vi "Set_Joint_State_Publlish_Rate.vi"(5 "node":string, 6 "error in":errorcluster, 9 "Publish Rate":u32) -> (0 "error out":errorcluster)   [LabVIEW 2013]
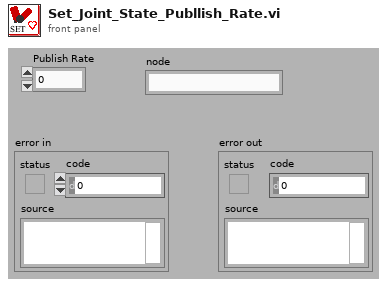
[diagram p1: front panel]
types:
  T1 = enum16{"big-endian, network order", "native, host order", "little-endian"}
  T2 = typedef "_ROSControl.ctl" = cluster{"topic port":u16, "Node":string, "topic":string, "type":string, "node port":u32, "error ":errorcluster, "Direction":T3, "APIs":string[]}
  T3 = typedef "_ROSDirection.ctl" = enum16{"Node", "Publisher", "Subscriber", "Service Client"}
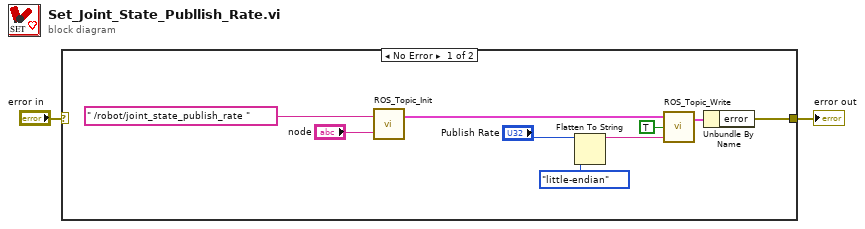
[diagram p0: block diagram]
diagram:
  n1 = case shown="No Error" "error in" {
    selector: "error in" -> [_ w12]
    tunnel: [w11 w12] -> w2
    frame No Error {
      n2 = call "ROS_Topic_Init.vi"("node"="node", "topic"=" /robot/joint_state_publish_rate ") -> ("ROS out"=w9:T2)  [unwired: 1 in]
      n3 = Flatten To String(anything="Publish Rate", byte order (0:big-endian, network order)=T1."little-endian") -> (data string=w5:string)  [unwired: 2 in, 2 out]
      n4 = call "ROS_Topic_Write.vi"("Msg in"=w5, "Continuous?"=TRUE, "ROS in"=w9) -> ("ROS out"=w8:T2)  [unwired: 1 in]
      n5 = Unbundle By Name(w8) -> ("error"=w11:errorcluster)
    }
    frame Error {
    }
  }
  "error out" <- w2
